vi "Test Listbox.vi"() -> ()   [LabVIEW 2020]
uses:
  Glyph/Listbox Icon Canvas/Listbox Icon Canvas.lvclass
  Canvas/Drawer .Net.lvclass
  LV Awesome/LV Awesome.lvclass
  Glyph/Font Settings/Font Settings.lvclass
  C:/Users/simon/Documents/LabView/LV Smybol/Canvas/Drawer .Net.lvclass
  C:/Users/simon/Documents/LabView/LV Smybol/Glyph Drawer/Glyph Drawer.lvclass
  C:/Users/simon/Documents/LabView/LV Smybol/Glyph/Listbox Icon Canvas/Listbox Icon Canvas.lvclass
  C:/Users/simon/Documents/LabView/LV Smybol/Glyph/Glyph Canvas/Glyph Canvas.lvclass
panel:
  in  "Listbox":i32(listbox)
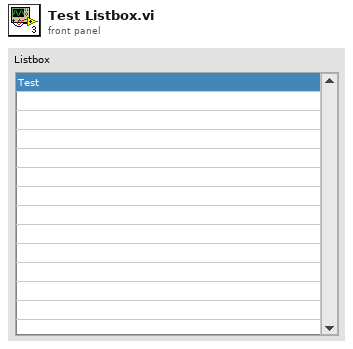
[diagram p1: front panel]
types:
  T1 = cluster{"Front":cluster{"Color":u32, "Alpha":u8}, "Back":cluster{"Color":u32, "Alpha":u8}}
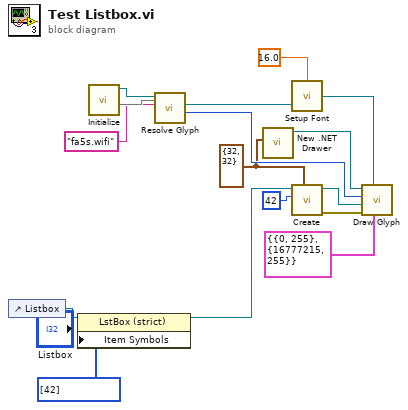
[diagram p0: block diagram]
diagram:
  w1 = cluster{"width":i32, "height":i32} {"width"=32, "height"=32} ("Size")
  n1 = control-ref of="Listbox"() -> (w4:refnum<vi>)
  n2 = property class="LstBox (strict)"(reference=w4, "Item Symbols"=i32[] [42]) -> (reference out=w2:refnum<vi>)  [unwired: 1 in, 1 out]
  n3 = call "Initialize.vi"() -> (1:w13, "LV Awesome"=w14:refnum<class "LV Awesome.lvclass">)  [unwired: 9 in, 1 out]
  n4 = call-dynamic "Resolve Glyph.vi"("Size"=w13, "Glyph Name"="fa5s.wifi", "LV-Awesome.lvlib:LV Awesome.lvclass"=w14) -> ("charcode"=w11:u32, "Font Settings out"=w9:refnum<class "Font Settings.lvclass">)  [unwired: 5 in, 2 out]
  n5 = call "New .NET Drawer.vi"(10:w1) -> ("Canvas out"=w15:refnum<class "Drawer .Net.lvclass">)  [unwired: 9 in, 1 out]
  n6 = call "Setup Font.vi"("Size"=16.0, "Font Path (System)"=w9) -> ("Font Settings out"=w10:refnum<class "Font Settings.lvclass">)  [unwired: 1 in]
  n7 = call "Create.vi"("Size"=w1, "Index (42)"=42, "Listbox"=w2) -> ("error out"=w5:errorcluster, "Listbox Icon Canvas out"=w6:refnum<class "Listbox Icon Canvas.lvclass">)  [unwired: 7 in]
  n8 = call-dynamic "Draw Glyph.vi"("Colors"=T1 {"Front"={"Color"=0, "Alpha"=255}, "Back"={"Color"=16777215, "Alpha"=255}}, "Font (System)"=w10, "error in (no error)"=w5, "Destination"=w6, "codepoint"=w11, "Canvas .Net in"=w15) -> ()  [unwired: 3 in, 3 out]
